vi "mtlb simx Query.vi"(0 "clientIDandSignalLengthAndTimeOutInMs":i32, 1 "retSignalValue":string, 5 "signalName":string, 7 "signalValue":string, 9 "retSignalName":string, 11 "error in (no error)":errorcluster, 12 "retSignalLength":i32) -> (3 "retSignalValue out":string, 4 "clientIDandSignalLengthAndTimeOutInMs out":i32, 6 "function return":i32, 14 "retSignalLength out":i32, 15 "error out":errorcluster)   [LabVIEW 2019, in "PXL_V-REP.lvlib"]
doc: "EXTAPI_DLLEXPORT simxInt mtlb_simxQuery(simxInt* clientIDandSignalLengthAndTimeOutInMs,const simxChar* signalName,const simxUChar* signalValue,const simxChar* retSignalName,simxUChar** retSignalValue,simxInt* retSignalLength);"
uses:
  PXL_V-REP.lvlib
  <userlib>/V-REP/remoteApi.dll
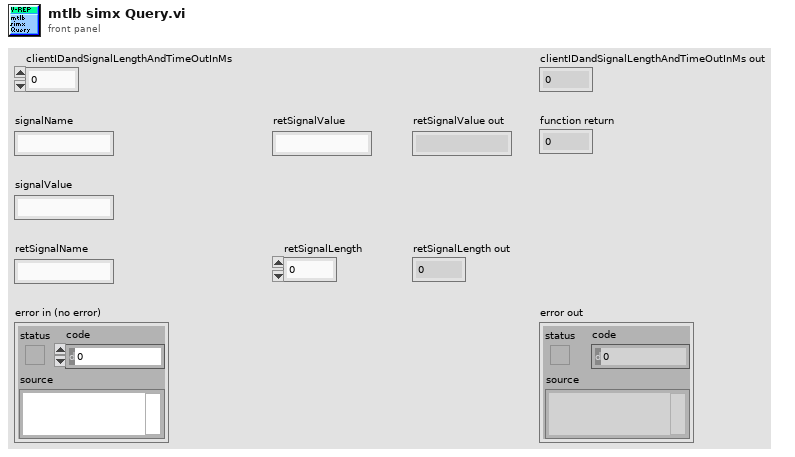
[diagram p1: front panel]
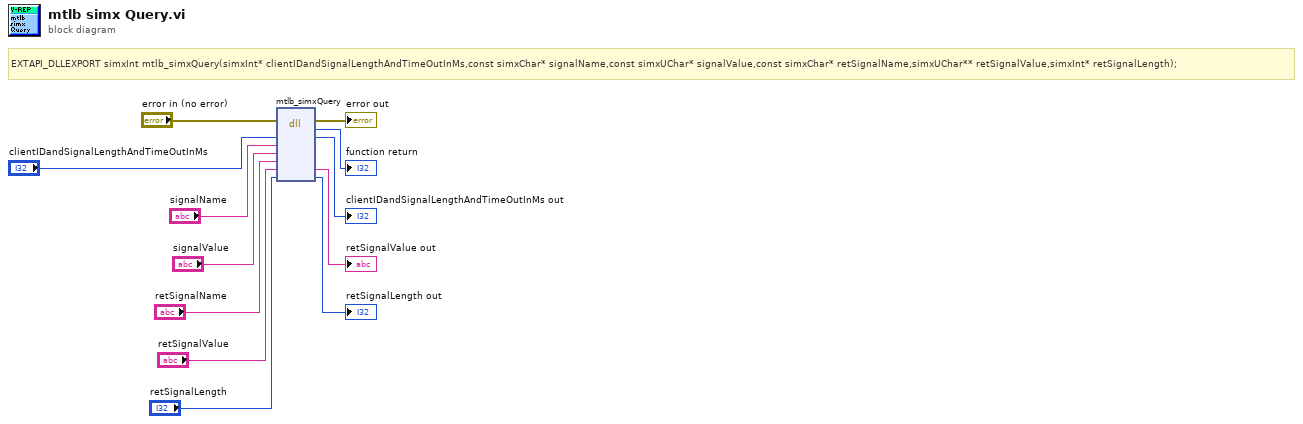
[diagram p0: block diagram]
diagram:
  # "EXTAPI_DLLEXPORT simxInt mtlb_simxQuery(simxInt* clientIDandSignalLengthAndTimeOutInMs,const simxChar* signalName,const simxUChar* signalValue,const simxChar* retSignalName,simxUChar** retSignalValue,simxInt* retSignalLength);"
  n1 = dll-call lib="C:/Program Files (x86)/National Instruments/LabVIEW 2019/user.lib/V-REP/remoteApi.*" fn="mtlb_simxQuery"(error in="error in (no error)", "clientIDandSignalLengthAndTimeOutInMs"="clientIDandSignalLengthAndTimeOutInMs", "signalName"="signalName", "signalValue"="signalValue", "retSignalName"="retSignalName", "retSignalValue"="retSignalValue", "retSignalLength"="retSignalLength") -> (error out=→"error out":errorcluster, →"function return":i32, "clientIDandSignalLengthAndTimeOutInMs"=→"clientIDandSignalLengthAndTimeOutInMs out":i32, "retSignalValue"=→"retSignalValue out":string, "retSignalLength"=→"retSignalLength out":i32)  [unwired: 5 in, 1 out]
